vi "Interpolate DBL.vi"() -> ()   [LabVIEW 2018]
panel:
  out "Current Value":dbl
  in  "Ending Value":dbl
  in  "Starting Value":dbl
  in  "Current Time":dbl
  in  "Duration":dbl
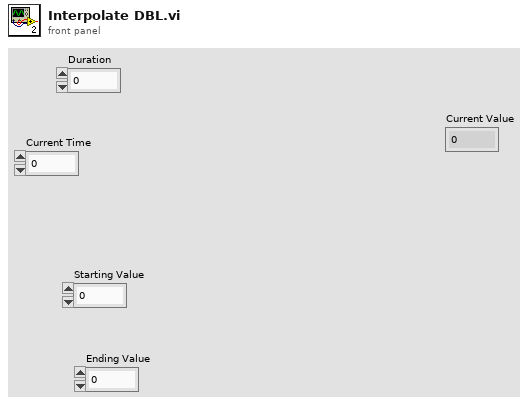
[diagram p1: front panel]
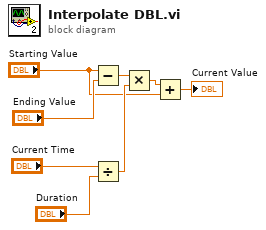
[diagram p0: block diagram]
diagram:
  n1 = Subtract(x="Starting Value", y="Ending Value") -> (x-y=w7:dbl)
  n2 = Divide(x="Current Time", y="Duration") -> (x/y=w4:dbl)
  n3 = Multiply(x=w7, y=w4) -> (x*y=w3:dbl)
  n4 = Add(x=w3, y="Starting Value") -> (x+y=→"Current Value":dbl)
